vi "Configure LXI Event Output.vi"(0 "VISA resource name":refnum<visa-resource-name>, 1 "Enable Event Output(T: Enable)":bool=TRUE, 2 "LXI Destination Host Names":string[](array[string]), 3 "LAN Identifiers":string[](array[string]), 5 "LXI Event (0: LAN0)":i32(ring) items=["LAN0", "LAN1", "LAN2", "LAN3", "LAN4", "LAN5", "LAN6", "LAN7"], 7 "LXI Event Source (0: WaitingForAcquireArm1)":i32(ring) items=["WaitingForAcquireArm1", "WaitingForTransitionArm1", "WaitingForAcquireArm2", "WaitingForTransitionArm2", "WaitingForAcquireTrigger1", "WaitingForTransitionTrigger1", "WaitingForAcquireTrigger2", "WaitingForTransitionTrigger2", "Measuring1", "Measuring2", "Settling1", "Settling2"], 9 "LXI Event Slope (0: Negative)":i32(ring) items=["Negative", "Positive"], 11 "error in (no error)":errorcluster, 12 "LXI Event Drive (0: Off)":i32(ring) items=["Off", "Normal", "Wired-OR"], 13 "LXI Destination Port Numbers":i32[](array[numeric])) -> (4 "VISA resource name out":refnum<visa-resource-name>, 15 "error out":errorcluster)   [LabVIEW 2020, in "Agilent B2900 Series.lvlib"]
doc: "Configures LXI output triggers for status change between idle-arm, arm-trigger or trigger-action layer. \nTo use LXI output triggers, please set output trigger signal to LAN first.\nCall Configure Trigger Output.vi to configure output trigger signal."
uses:
  Agilent B2900 Series.lvlib
panel:
  # "LXI Event Destination"
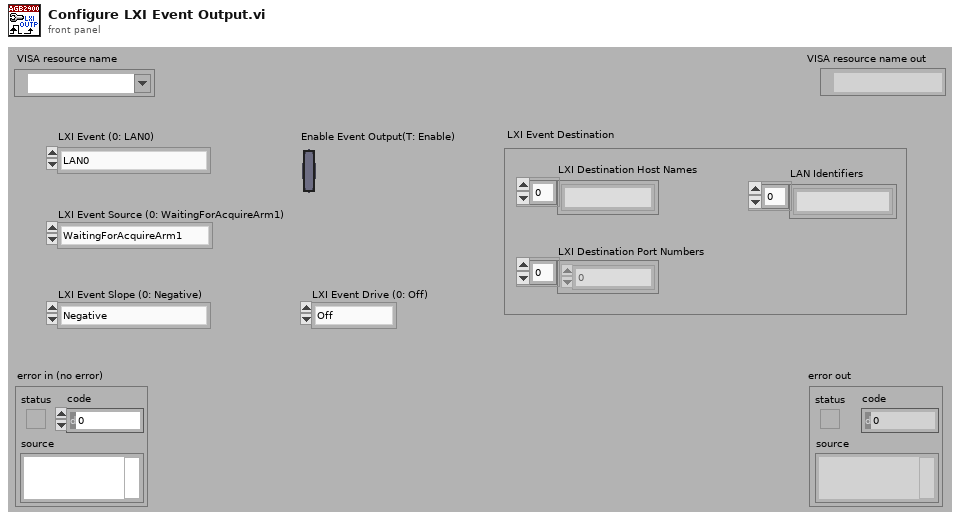
[diagram p1: front panel]
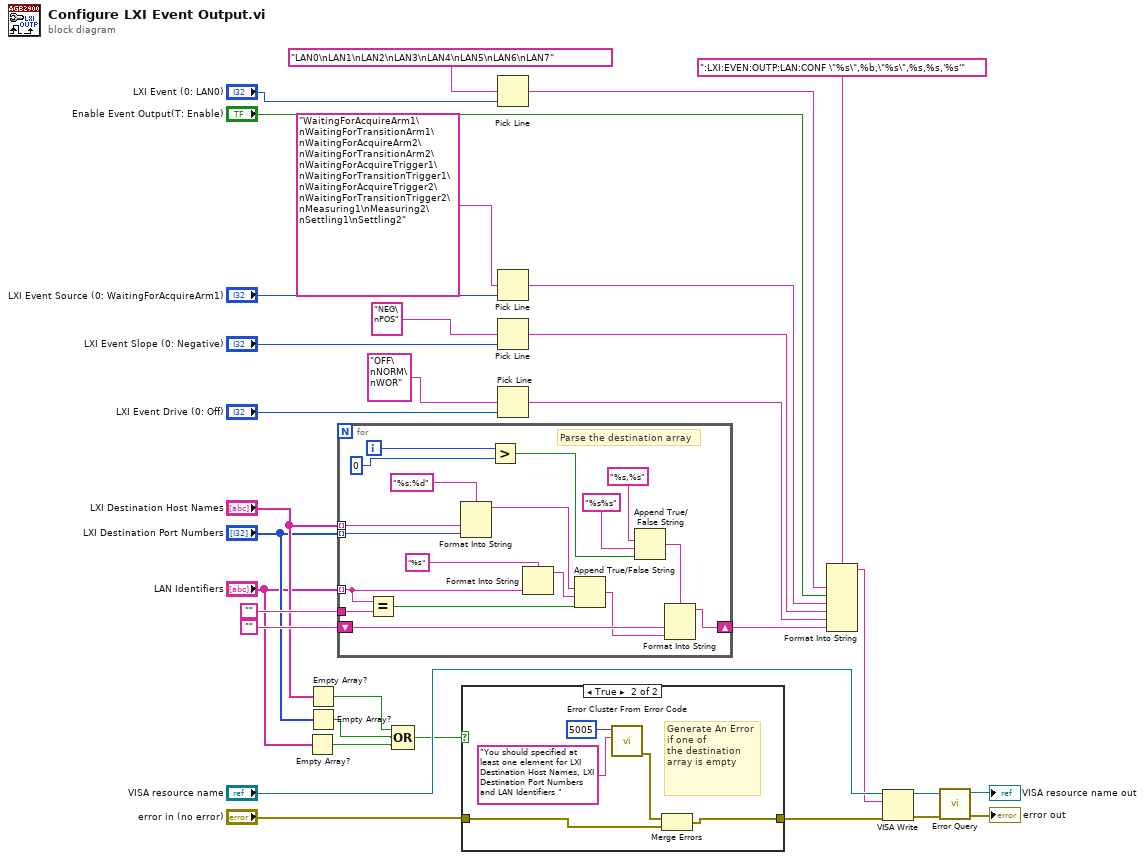
[diagram p0: block diagram]
diagram:
  n1 = Empty Array?(array="LAN Identifiers") -> (empty?=w5:bool)
  n2 = Empty Array?(array="LXI Destination Host Names") -> (empty?=w7:bool)
  n3 = Empty Array?(array="LXI Destination Port Numbers") -> (empty?=w6:bool)
  n4 = for {
    tunnel: "LXI Destination Host Names" -> [w49] mode=indexing
    tunnel: "LXI Destination Port Numbers" -> [w48] mode=indexing
    tunnel: "" ("Empty String Constant") -> [w47]
    tunnel: "LAN Identifiers" -> [w45] mode=indexing
    shift-right: [w35] -> w11
    shift-left: "" ("Empty String Constant") -> [w37]
    i -> [w34]
    # "Parse the destination array"
    n5 = Equal?(x=w45, y=w47) -> (x = y?=w41:bool)
    n6 = Format Into String(format string="%s:%d", w49, w48) -> (resulting string=w33:string)  [unwired: 2 in, 1 out]
    n7 = Greater?(x=w34, y=0) -> (0:w43:bool)
    n8 = Format Into String(format string="%s", w45) -> (resulting string=w42:string)  [unwired: 2 in, 1 out]
    n9 = Append True/False String(1:w41, 2:w42, 3:w33) -> (0:w36:string)  [unwired: 1 in]
    n10 = Append True/False String(1:w43, 2:"%s%s" ("false string"), 3:"%s,%s" ("true string")) -> (0:w38:string)  [unwired: 1 in]
    n11 = Format Into String(format string=w38, w37, w36) -> (resulting string=w35:string)  [unwired: 2 in, 1 out]
  }
  n12 = Compound Arithmetic op=OR(w7, w6, w5) -> (w8:bool)
  n13 = case shown="True" w8 {
    tunnel: [w51 w56] -> w10
    tunnel: "error in (no error)" -> [w51 w54]
    frame False {
    }
    frame True {
      # "Generate An Error if one of\nthe destination array is empty"
      n14 = call <vilib>:"Error Cluster From Error Code.vi"("error message (\"\")"="You should specified at least one element for LXI Destination Host Names, LXI Destination Port Numbers and LAN Identifiers " ("error message (\"\")"), "error code (0)"=5005) -> ("error out"=w55:errorcluster)  [unwired: 7 in]
      n15 = Merge Errors(w55, w54) -> (w56:errorcluster)
    }
  }
  n16 = Pick Line(multi-line string="LAN0\nLAN1\nLAN2\nLAN3\nLAN4\nLAN5\nLAN6\nLAN7", line index="LXI Event (0: LAN0)") -> (output string=w29:string)  [unwired: 1 in]
  n17 = Pick Line(multi-line string="WaitingForAcquireArm1\nWaitingForTransitionArm1\nWaitingForAcquireArm2\nWaitingForTransitionArm2\nWaitingForAcquireTrigger1\nWaitingForTransitionTrigger1\nWaitingForAcquireTrigger2\nWaitingForTransitionTrigger2\nMeasuring1\nMeasuring2\nSettling1\nSettling2", line index="LXI Event Source (0: WaitingForAcquireArm1)") -> (output string=w26:string)  [unwired: 1 in]
  n18 = Pick Line(multi-line string="NEG\nPOS", line index="LXI Event Slope (0: Negative)") -> (output string=w23:string)  [unwired: 1 in]
  n19 = Pick Line(multi-line string="OFF\nNORM\nWOR", line index="LXI Event Drive (0: Off)") -> (output string=w20:string)  [unwired: 1 in]
  n20 = Format Into String(format string=":LXI:EVEN:OUTP:LAN:CONF \"%s\",%b,\"%s\",%s,%s,'%s'", w29, "Enable Event Output(T: Enable)", w26, w23, w20, w11) -> (resulting string=w18:string)  [unwired: 2 in, 1 out]
  n21 = VISA Write(VISA resource name="VISA resource name", write buffer=w18, error in (no error)=w10) -> (VISA resource name out=w17:refnum<visa-resource-name>, error out=w16:errorcluster)  [unwired: 1 out]
  n22 = call "Error Query.vi"("error in (no error)"=w16, "VISA resource name"=w17) -> ("error out"=→"error out":errorcluster, "VISA resource name out"=→"VISA resource name out":refnum<visa-resource-name>)  [unwired: 6 in, 2 out]
